vi "iXonImage.vi"() -> ()   [LabVIEW 2009]
uses:
  C/Program Files (x86)/National Instruments/LabVIEW 2015/user.lib/atmcd32d.llb/Shutter_type typedef.ctl
panel:
  out "Intensity Graph":i32[][](graph)
  out "Detector Y Pixels":i32
  in  "Shutter Trigger":T1
  in  "Time to open or\nclose shutter (ms):":i32
  in  "Shut Down":bool
  in  "Start Acquisition":bool
  out "Return  from Get Acquired Data":u32
  out "Detector X Pixels":i32
  out "Return from GetStatus":u32
  out "Return from Start Acquisition":u32
  out "Return from CheckTimings Exposure":u32
  out "Calculated Exposure Value":sgl format="%.2f"
  in  "Exposure Time (secs)":sgl format="%.2f"
  out "Return from Initialize":u32
  in  "Trigger":u32(ring) items=["Internal", "External"]
  # "Status"
  # "Acquisition Mode: Single Scan\nReadout Mode: Full Resolution\nImage"
  # "Shutter Trigger"
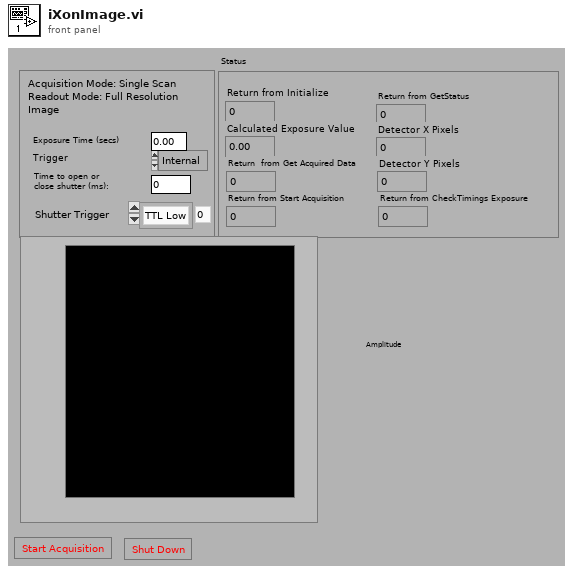
[diagram p1: front panel]
types:
  T1 = typedef "Shutter_type typedef.ctl" = enum16{"TTL Low", "TTL High"}
  T2 = typedef "Error Code Enum typedef.ctl" = enum32{"N/A (0)", "DRV_ERROR_CODES", "DRV_SUCCESS", "DRV_VXDNOTINSTALLED", "DRV_ERROR_SCAN", "DRV_ERROR_CHECK_SUM", "DRV_ERROR_FILELOAD", "DRV_UNKNOWN_FUNC", "DRV_ERROR_VXD_INIT", "DRV_ERROR_ADDRESS", "DRV_ERROR_PAGELOCK", "DRV_ERROR_PAGEUNLOCK", "DRV_ERROR_BOARDTEST", "DRV_ERROR_ACK", "DRV_ERROR_UP_FIFO", "DRV_ERROR_PATTERN", "N/A (16)", "DRV_ACQUISITION_ERRORS", "DRV_ACQ_BUFFER", "DRV_ACQ_DOWNFIFO_FULL", "DRV_PROC_UNKONWN_INSTRUCTION", "DRV_ILLEGAL_OP_CODE", "DRV_KINETIC_TIME_NOT_MET", "DRV_ACCUM_TIME_NOT_MET", "DRV_NO_NEW_DATA", "N/A (25)", "DRV_SPOOLERROR", "N/A (27)", "N/A (28)", "N/A (29)", "N/A (30)", "N/A (31)", "N/A (32)", "DRV_TEMPERATURE_CODES", "DRV_TEMPERATURE_OFF", "DRV_TEMPERATURE_NOT_STABILIZED", "DRV_TEMPERATURE_STABILIZED", "DRV_TEMPERATURE_NOT_REACHED", "DRV_TEMPERATURE_OUT_RANGE", "DRV_TEMPERATURE_NOT_SUPPORTED", "DRV_TEMPERATURE_DRIFT", "N/A (41)", "N/A (42)", "N/A (43)", "N/A (44)", "N/A (45)", "N/A (46)", "N/A (47)", "N/A (48)", "DRV_GENERAL_ERRORS", "DRV_INVALID_AUX", "DRV_COF_NOTLOADED", "DRV_FPGAPROG", "DRV_FLEXERROR", "DRV_GPIBERROR", "N/A (55)", "N/A (56)", "N/A (57)", "N/A (58)", "N/A (59)", "N/A (60)", "N/A (61)", "N/A (62)", "N/A (63)", "DRV_DATATYPE", "DRV_DRIVER_ERRORS", "DRV_P1INVALID", "DRV_P2INVALID", "DRV_P3INVALID", "DRV_P4INVALID", "DRV_INIERROR", "DRV_COFERROR", "DRV_ACQUIRING", "DRV_IDLE", "DRV_TEMPCYCLE", "DRV_NOT_INITIALIZED", "DRV_P5INVALID", "DRV_P6INVALID", "DRV_INVALID_MODE", "DRV_INVALID_FILTER", "DRV_I2CERRORS", "DRV_I2CDEVNOTFOUND", "DRV_I2CTIMEOUT", "DRV_P7INVALID", "N/A (84)", "N/A (85)", "N/A (86)", "N/A (87)", "N/A (88)", "N/A (89)", "DRV_IOCERROR", "DRV_VRMVERSIONERROR"}
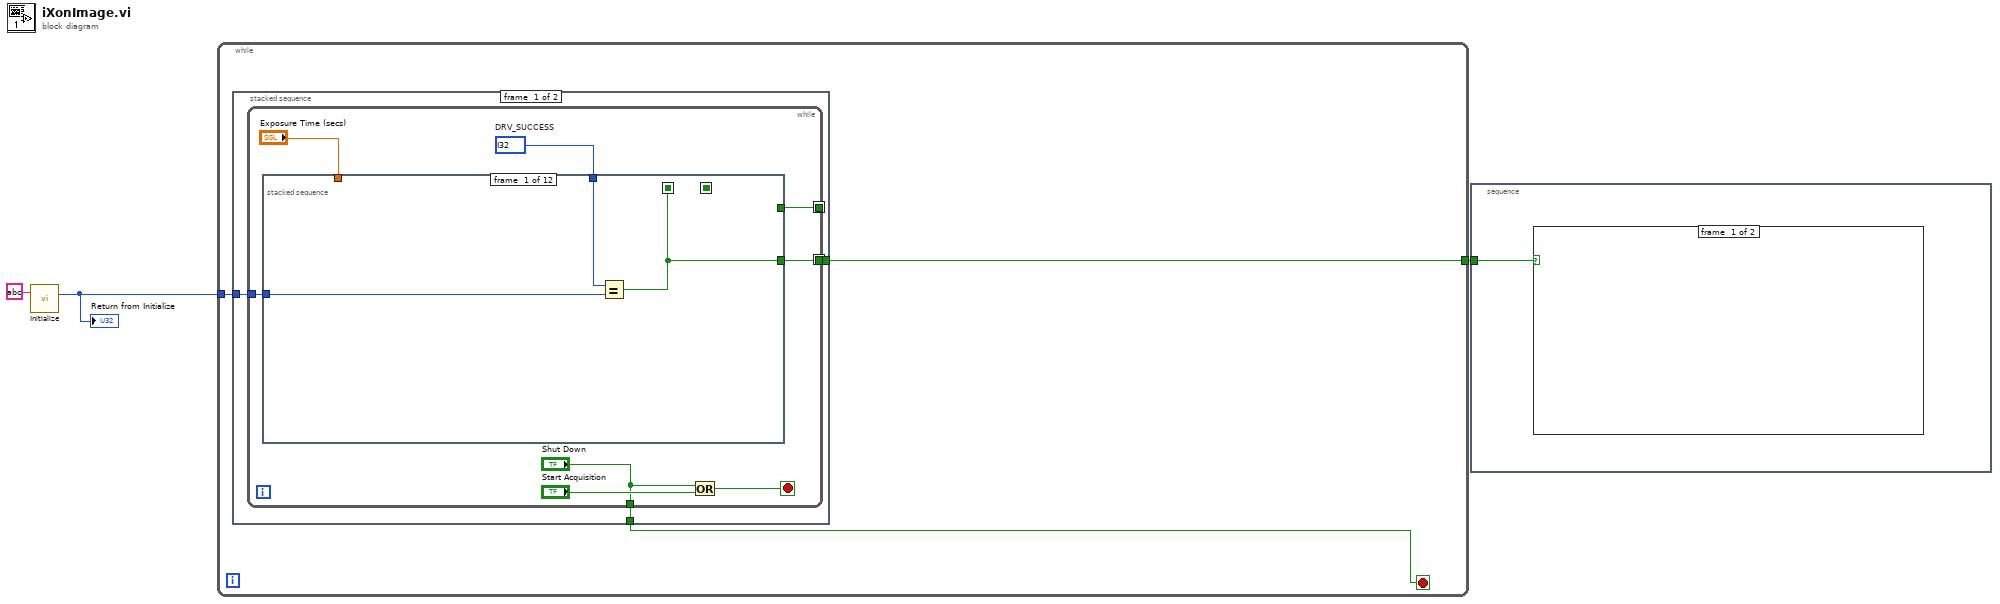
[diagram p0: block diagram]
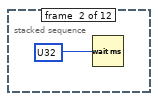
[diagram p2: hidden frame]
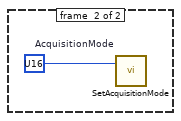
[diagram p4: hidden frame]
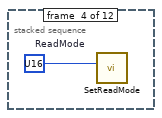
[diagram p5: hidden frame]
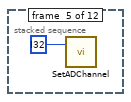
[diagram p6: hidden frame]
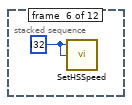
[diagram p7: hidden frame]
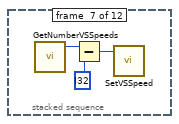
[diagram p8: hidden frame]
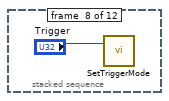
[diagram p9: hidden frame]
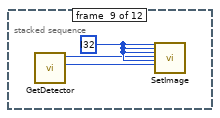
[diagram p10: hidden frame]
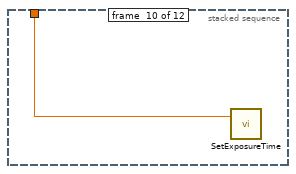
[diagram p11: hidden frame]
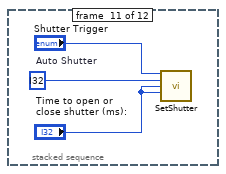
[diagram p12: hidden frame]
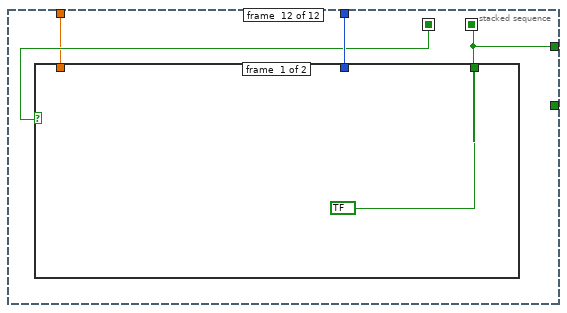
[diagram p13: hidden frame]
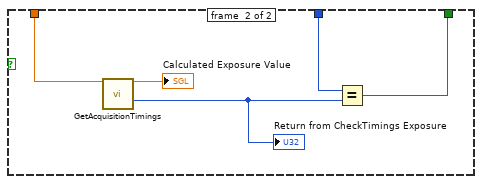
[diagram p14: hidden frame]
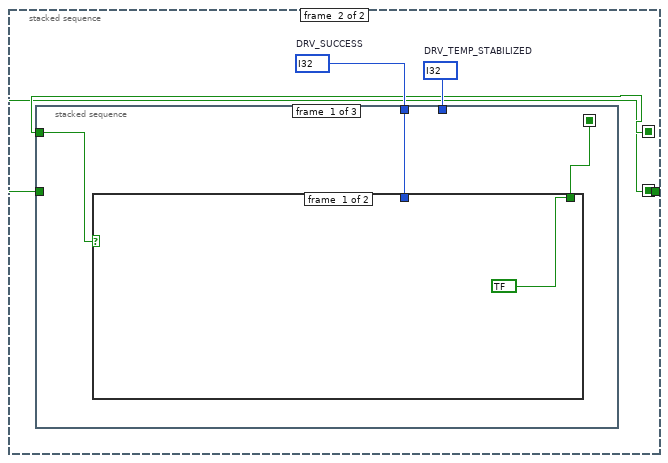
[diagram p15: hidden frame]
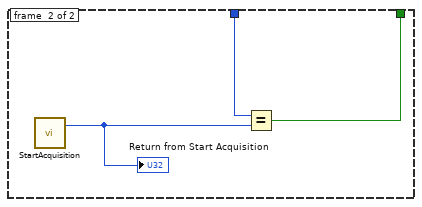
[diagram p16: hidden frame]
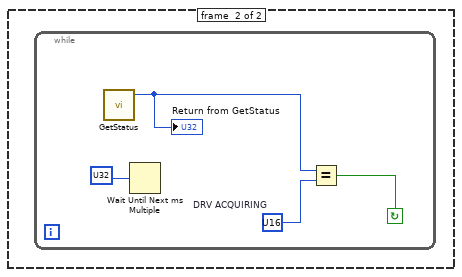
[diagram p18: hidden frame]
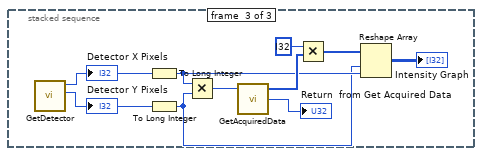
[diagram p19: hidden frame]
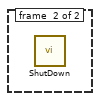
[diagram p20: hidden frame]
diagram:
  n1 = call "Initialize.vi"("directory (\"\")"=string ? ("directory (\"\")")) -> ("DLL error code"=w2:u32)  [unwired: 1 in, 1 out]
  "Return from Initialize" <- w2
  n2 = while {
    tunnel: w2 -> [w6]
    tunnel: [w5] -> w1
    stop <- w4 stop-if-true
    n3 = stacked-sequence {
      seq-local: [w9 _] -> [_ w50]
      seq-local: [w8 _] -> [_ w49]
      tunnel: w6 -> [w10 _]
      tunnel: [w7 _] -> w4
      tunnel: [_ w49] -> w5
      frame #0 {
        n4 = while {
          tunnel: w10 -> [w16]
          tunnel: [w15] -> w9
          tunnel: [w14] -> w8
          tunnel: ["Shut Down"] -> w7
          stop <- w12 stop-if-true
          w17 = i32 ?  # DRV_SUCCESS
          n5 = stacked-sequence {
            seq-local: [w19 _ _ _ _ _ _ _ _ _ _ _] -> [_ _ w23 _ _ _ _ _ _ _ _ w41]
            seq-local: [_ _ _ _ _ _ _ _ _ _ _ w39] -> [_ _ _ _ _ _ _ _ _ _ _ _]
            tunnel: "Exposure Time (secs)" -> [_ _ _ _ _ _ _ _ _ w35 _ w40]
            tunnel: w17 -> [w21 _ _ _ _ _ _ _ _ _ _ w42]
            tunnel: w16 -> [w20 _ _ _ _ _ _ _ _ _ _ _]
            tunnel: [_ _ _ _ _ _ _ _ _ _ _ w39] -> w15
            tunnel: [w19 _ _ _ _ _ _ _ _ _ _ _] -> w14
            frame #0 {
              n6 = Equal?(x=w21, y=w20) -> (x = y?=w19:bool)
            }
            frame #1 {
              n7 = Wait (ms)(milliseconds to wait=u32 ?) -> ()  [unwired: 1 out]
            }
            frame #2 {
              n8 = case shown="True" w23 {
                frame #0 {
                }
                frame #1 {
                  w24 = u16 ?  # AcquisitionMode
                  n9 = call "SetAcquisitionMode.vi"("mode"=w24) -> ()  [unwired: 1 in, 2 out]
                }
              }
            }
            frame #3 {
              w25 = u16 ?  # ReadMode
              n10 = call "SetReadMode.vi"("mode"=w25) -> ()  [unwired: 1 in, 2 out]
            }
            frame #4 {
              n11 = call "SetADChannel.vi"("channel"=i32 ?) -> ()  [unwired: 1 in, 2 out]
            }
            frame #5 {
              w27 = i32 ?
              n12 = call "SetHSSpeed.vi"("index"=w27, "type"=w27) -> ()  [unwired: 2 in, 2 out]
            }
            frame #6 {
              n13 = call "GetNumberVSSpeeds.vi"() -> ("number"=w30:i32)  [unwired: 3 in, 2 out]
              n14 = Subtract(x=w30, y=i32 ?) -> (x-y=w28:i32)
              n15 = call "SetVSSpeed.vi"("index"=w28) -> ()  [unwired: 1 in, 2 out]
            }
            frame #7 {
              n16 = call "SetTriggerMode.vi"("mode"="Trigger") -> ()  [unwired: 1 in, 2 out]
            }
            frame #8 {
              w34 = i32 ? ("hbin")
              n17 = call "GetDetector.vi"() -> ("ypixels"=w32:i32, "xpixels"=w33:i32)  [unwired: 4 in, 2 out]
              n18 = call "SetImage.vi"("hbin"=w34, "vbin"=w34, "hstart"=w34, "hend"=w33, "vstart"=w34, "vend"=w32) -> ()  [unwired: 20 in, 2 out]
            }
            frame #9 {
              n19 = call "SetExposureTime.vi"("time"=w35) -> ()  [unwired: 1 in, 2 out]
            }
            frame #10 {
              w37 = i32 ?  # Auto Shutter
              n20 = call "SetShutter.vi"("type"="Shutter Trigger", "mode"=w37, "closingtime"="Time to open or\nclose shutter (ms):", "openingtime"="Time to open or\nclose shutter (ms):") -> ()  [unwired: 10 in, 2 out]
            }
            frame #11 {
              n21 = case shown="True" w41 {
                tunnel: w42 -> [_ w45]
                tunnel: [bool ? w48] -> w39
                tunnel: w40 -> [_ w46]
                frame #0 {
                }
                frame #1 {
                  n22 = call "GetAcquisitionTimings.vi"("exposure input"=w46) -> ("exposure"=→"Calculated Exposure Value":sgl, "DLL error code"=w44:u32)  [unwired: 10 in, 3 out]
                  "Return from CheckTimings Exposure" <- w44
                  n23 = Equal?(x=w45, y=w44) -> (x = y?=w48:bool)
                }
              }
            }
          }
          n24 = Or(x="Shut Down", y="Start Acquisition") -> (x .or. y?=w12:bool)
        }
      }
      frame #1 {
        w51 = i32 ?  # DRV_TEMP_STABILIZED
        w52 = i32 ?  # DRV_SUCCESS
        n25 = stacked-sequence {
          seq-local: [w54 _ _] -> [_ w60 _]
          tunnel: w52 -> [w55 _ _]
          tunnel: w51 -> [_ _ _]
          tunnel: w50 -> [w53 _ _]
          tunnel: w49 -> [_ _ _]
          frame #0 {
            n26 = case shown="True" w53 {
              tunnel: [bool ? w59] -> w54
              tunnel: w55 -> [_ w58]
              frame #0 {
              }
              frame #1 {
                n27 = call "StartAcquisition.vi"() -> ("DLL error code"=w57:u32)  [unwired: 2 in, 1 out]
                "Return from Start Acquisition" <- w57
                n28 = Equal?(x=w58, y=w57) -> (x = y?=w59:bool)
              }
            }
          }
          frame #1 {
            n29 = case shown="True" w60 {
              frame #0 {
              }
              frame #1 {
                n30 = while {
                  stop <- w63 continue-if-true
                  w62 = u16 ?  # DRV ACQUIRING
                  n31 = call "GetStatus.vi"() -> ("status"=w61:T2)  [unwired: 3 in, 2 out]
                  "Return from GetStatus" <- w61
                  n32 = Wait Until Next ms Multiple(millisecond multiple=u32 ?) -> ()  [unwired: 1 out]
                  n33 = Equal?(x=w61, y=w62) -> (x = y?=w63:bool)
                }
              }
            }
          }
          frame #2 {
            n34 = call "GetDetector.vi"() -> ("ypixels"=w71:i32, "xpixels"=w74:i32)  [unwired: 4 in, 2 out]
            "Detector X Pixels" <- w74
            "Detector Y Pixels" <- w71
            n35 = To Long Integer(number=w74) -> (32bit integer=w66:i32)
            n36 = To Long Integer(number=w71) -> (32bit integer=w65:i32)
            n37 = Multiply(x=w66, y=w65) -> (x*y=w72:i32)
            n38 = call "GetAcquiredData.vi"("size"=w72) -> ("DLL error code"=→"Return  from Get Acquired Data":u32, "array"=w69:i32[])  [unwired: 2 in, 1 out]
            n39 = Multiply(x=i32 ?, y=w69) -> (x*y=w68:i32[])
            n40 = Reshape Array(w68, w65, w66) -> (→"Intensity Graph":i32[][])
          }
        }
      }
    }
  }
  n41 = stacked-sequence {
    tunnel: w1 -> [w75]
    frame #0 {
      n42 = case shown="True" w75 {
        frame #0 {
        }
        frame #1 {
          n43 = call "ShutDown.vi"() -> ()  [unwired: 2 in, 2 out]
        }
      }
    }
  }
